vi "Queue Transport.vi"() -> (2 "Transport":refnum<class "Transport.lvclass">)   [LabVIEW 2025, in "jettl.lvlib" / "Transport.lvlib"]
uses:
  Transport.lvlib
  Queue Transport/Queue Transport.lvclass
  C:/git/jettl/src/jettl/jettl/Transport/Queue Transport/Queue Transport.lvclass
  C:/git/jettl/src/jettl/jettl/Transport/Transport/Transport.lvclass
  Transport/Transport.lvclass
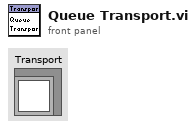
[diagram p1: front panel]
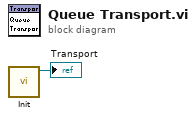
[diagram p0: block diagram]
diagram:
  n1 = call "Init.vi"() -> ("Queue Transport out"=→"Transport":refnum<class "Queue Transport.lvclass">)  [unwired: 11 in]
